vi "Parsing Data.vi"(8 "error in (no error)":errorcluster caption="entrée d'erreur (pas d'erreur)", 11 "Parsing Enocean (Default) en entrée":refnum<class "Parsing Data Enocean (Default).lvclass">) -> (0 "error out":errorcluster caption="sortie d'erreur", 3 "Parsing Enocean (Default) en sortie":refnum<class "Parsing Data Enocean (Default).lvclass">)   [LabVIEW 2020, in "Library Instrument & Equipement.lvlib" / "Library UART.lvlib" / "Parsing Data Enocean (Default).lvclass"]
uses:
  Parsing Data Enocean (Default).lvclass
  C:/Users/ngarcin/OneDrive - Altyor/Standard TB/Class/UART/UART (Default)/Parsing Data (Default)/Parsing Data (Default).lvclass
  Parsing Data Enocean (Default).lvclass/Parsing Data Enocean (Default).ctl
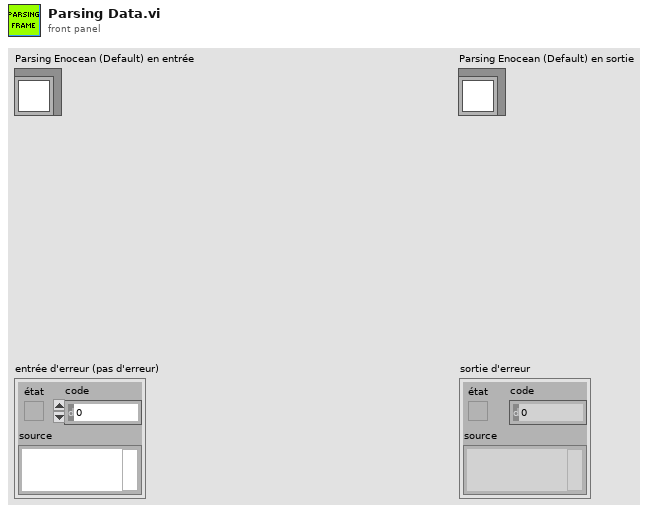
[diagram p1: front panel]
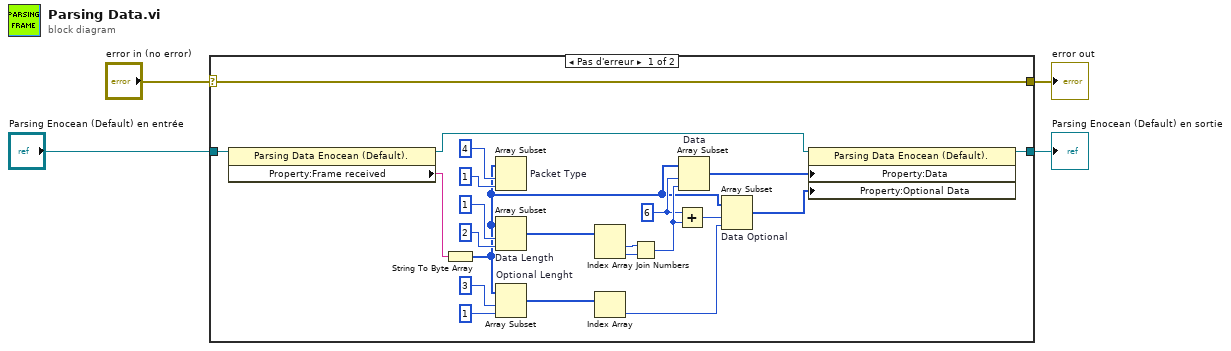
[diagram p0: block diagram]
diagram:
  n1 = case shown="Pas d'erreur" "error in (no error)" {
    selector: "error in (no error)" -> [w26 w28]
    tunnel: [w26 w28] -> w3
    tunnel: [w18 w27] -> w1
    tunnel: "Parsing Enocean (Default) en entrée" -> [w25 w27]
    frame No Error {
      w8 = 6 ("indice")
      n2 = property class="Parsing Data Enocean (Default)."(reference=w25) -> (reference out=w24:refnum<class "Parsing Data Enocean (Default).lvclass">, "Property:Frame received"=w19:string)  [unwired: 1 in, 1 out]
      n3 = String To Byte Array(string=w19) -> (unsigned byte array=w5:u8[])
      n4 = Array Subset "Packet Type"(array=w5, index=4 ("indice"), length=1 ("longueur")) -> ()  [unwired: 1 out]
      n5 = Array Subset "Data Length"(array=w5, index=1 ("indice"), length=2 ("longueur")) -> (w15:u8[])
      n6 = Array Subset "Optional Lenght"(array=w5, index=3 ("indice"), length=1 ("longueur")) -> (w10:u8[])
      n7 = Index Array(array=w15) -> (element #1=w17:u8, element #2=w16:u8)  [unwired: 2 in]
      n8 = Index Array(array=w10) -> (element=w9:u8)  [unwired: 1 in]
      n9 = Join Numbers(hi=w17, lo=w16) -> ((hi.lo)=w12:u16)
      n10 = Add(x=w8, y=w12) -> (x+y=w13:i32)
      n11 = Array Subset "Data"(array=w5, index=w8, length=w12) -> (w14:u8[])
      n12 = Array Subset "Data Optional"(array=w5, index=w13, length=w9) -> (w11:u8[])
      n13 = property class="Parsing Data Enocean (Default)."(reference=w24, "Property:Data"=w14, "Property:Optional Data"=w11) -> (reference out=w18:refnum<class "Parsing Data Enocean (Default).lvclass">)  [unwired: 1 in, 1 out]
    }
    frame Error {
    }
  }
  "error out" <- w3
  "Parsing Enocean (Default) en sortie" <- w1
